vi "Create IQ pulse.vi"() -> ()   [LabVIEW 2019]
uses:
  <vilib>/Analysis/1siggen.llb/Ramp Pattern by Samples.vi
  <vilib>/Analysis/NI_AALBase.lvlib
panel:
  in  "fs":dbl format="%#_6p"
  in  "duration":dbl format="%#_6p"
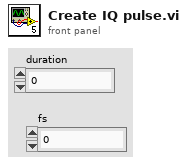
[diagram p1: front panel]
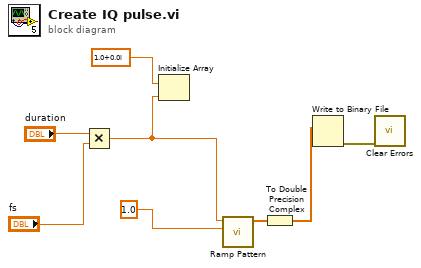
[diagram p0: block diagram]
diagram:
  n1 = Multiply(x="duration", y="fs") -> (x*y=w4:dbl)
  n2 = Initialize Array(cdb 1.0+0.0i, w4) -> ()  [unwired: 1 out]
  n3 = call-poly <vilib>:"Ramp Pattern.vi"("end"=1.0, "samples"=w4) -> ("Ramp Pattern"=w2:dbl[])  [unwired: 8 in, 1 out]
  n4 = To Double Precision Complex(1:w2) -> (0:w1:cdb[])
  n5 = Write to Binary File(data=w1) -> (error out=w5:errorcluster)  [unwired: 5 in, 2 out]
  n6 = call <vilib>:"Clear Errors.vi"("error in (no error)"=w5) -> ()  [unwired: 5 in, 2 out]
